vi "ExecutionWaitTime.vi"(8 "error in (no error)":errorcluster, 9 "Channel":i32, 10 "New Value":dbl, 11 "CaenHVSupply in":refnum<class "BK_PowerSupply.lvclass">) -> (0 "error out":errorcluster, 1 "Time to wait (ms)":dbl, 3 "CaenHVSupply out":refnum<class "BK_PowerSupply.lvclass">)   [LabVIEW 2020, in "BK_PowerSupply.lvclass"]
uses:
  BK_PowerSupply.lvclass
  BK_PowerSupply.lvclass/BK_PowerSupply.ctl
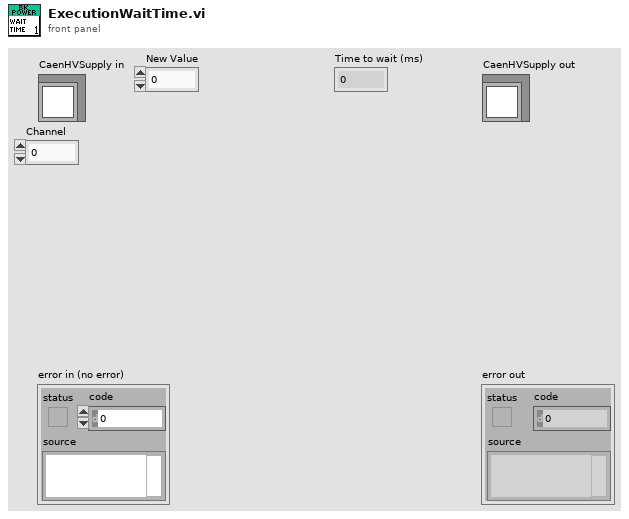
[diagram p1: front panel]
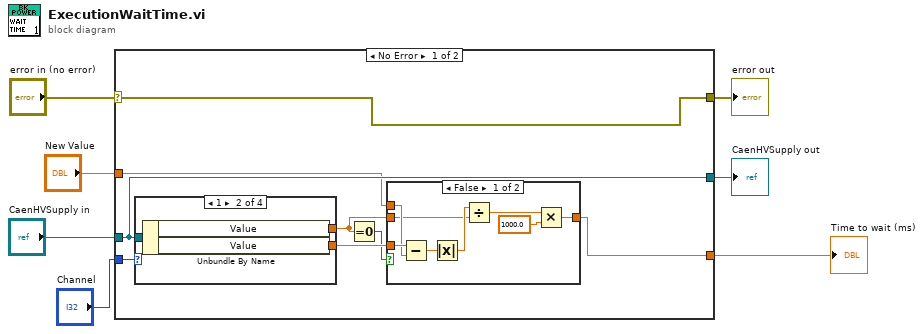
[diagram p0: block diagram]
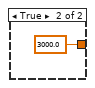
[diagram p2: hidden frame]
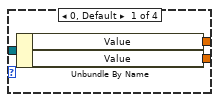
[diagram p3: hidden frame]
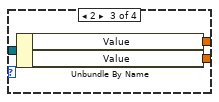
[diagram p4: hidden frame]
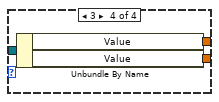
[diagram p5: hidden frame]
diagram:
  n1 = case shown="No Error" "error in (no error)" {
    selector: "error in (no error)" -> [w8 w38]
    tunnel: [w8 w38] -> w6
    tunnel: [w15 w37] -> w4
    tunnel: "CaenHVSupply in" -> [w15 w37]
    tunnel: "Channel" -> [w14 _]
    tunnel: "New Value" -> [w12 _]
    tunnel: [w9 _] -> w1
    frame No Error {
      n2 = case shown="1" w14 {
        tunnel: [w27 w30 w33 w36] -> w11
        tunnel: w15 -> [w25 w28 w31 w35]
        tunnel: [w26 w29 w32 w34] -> w13
        frame 0, Default {
          n3 = Unbundle By Name(w25) -> ("Value"=w27:dbl, "Value"=w26:dbl)
        }
        frame 1 {
          n4 = Unbundle By Name(w28) -> ("Value"=w30:dbl, "Value"=w29:dbl)
        }
        frame 2 {
          n5 = Unbundle By Name(w31) -> ("Value"=w33:dbl, "Value"=w32:dbl)
        }
        frame 3 {
          n6 = Unbundle By Name(w35) -> ("Value"=w36:dbl, "Value"=w34:dbl)
        }
      }
      n7 = Equal To 0?(x=w11) -> (x = 0?=w10:bool)
      n8 = case shown="False" w10 {
        tunnel: w13 -> [w23 _]
        tunnel: w12 -> [w22 _]
        tunnel: w11 -> [w19 _]
        tunnel: [w16 3000.0] -> w9
        frame False {
          n9 = Subtract(x=w23, y=w22) -> (x-y=w21:dbl)
          n10 = Absolute Value(x=w21) -> (abs(x)=w20:dbl)
          n11 = Divide(x=w20, y=w19) -> (x/y=w18:dbl)
          n12 = Multiply(x=w18, y=1000.0) -> (x*y=w16:dbl)
        }
        frame True {
        }
      }
    }
    frame Error {
    }
  }
  "error out" <- w6
  "CaenHVSupply out" <- w4
  "Time to wait (ms)" <- w1
